vi "GV rescan galvo delay.vi"() -> ()   [LabVIEW 2017]
panel:
  out "RescanGalvoDelay_tick":u16
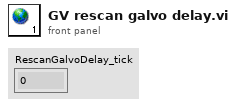
[diagram p1: front panel]
diagram:
